vi "TetrisLV.vi"(11 "Board Size":T1={"X"=10, "Y"=20}) -> ()   [LabVIEW 2017]
uses:
  Controls/Coordinates.ctl
  Controls/Moves.ctl
  Game Board_class/Game Board.lvclass
  Wall_class/Wall.lvclass
  Piece of Bricks_class/Piece of Bricks.lvclass
panel:
  in  "Sounds On/Off":bool caption="Sounds"
  in  "Music On/Off":bool caption="Music"
  in  "Tableau":u32[][](array[colorbox])
  in  "Bouton Stop":bool
  out "Screen":u32[][](array[colorbox])
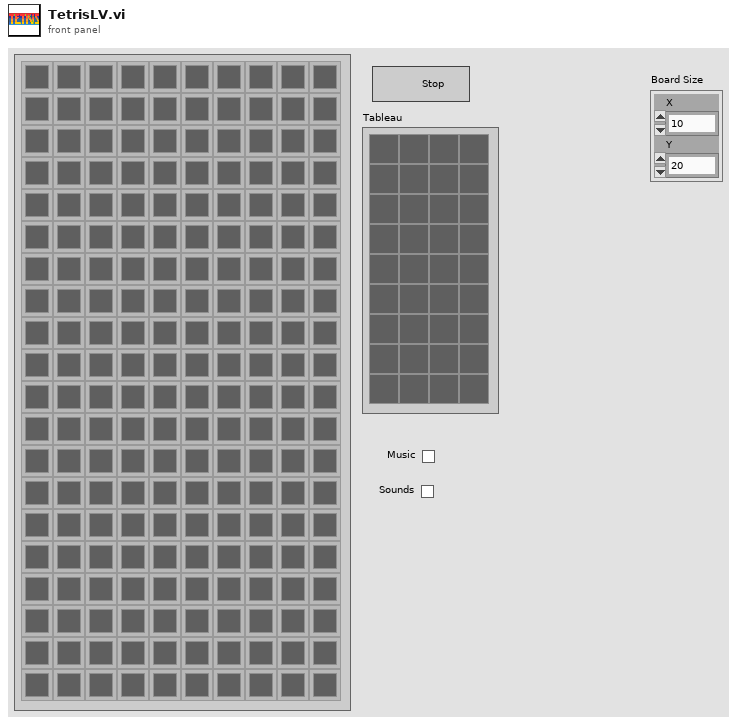
[diagram p1: front panel]
types:
  T1 = typedef "Coordinates.ctl" = cluster{"X":i32, "Y":i32}
  T2 = typedef "Moves.ctl" = enum16{"None", "Right", "Left", "Step Down", "Go Down", "90 Clockwise", "90 Anti-Clockwise"}
  T3 = enum32{"Invalid", "Standard", "Closed", "Hidden", "Minimized", "Maximized"}
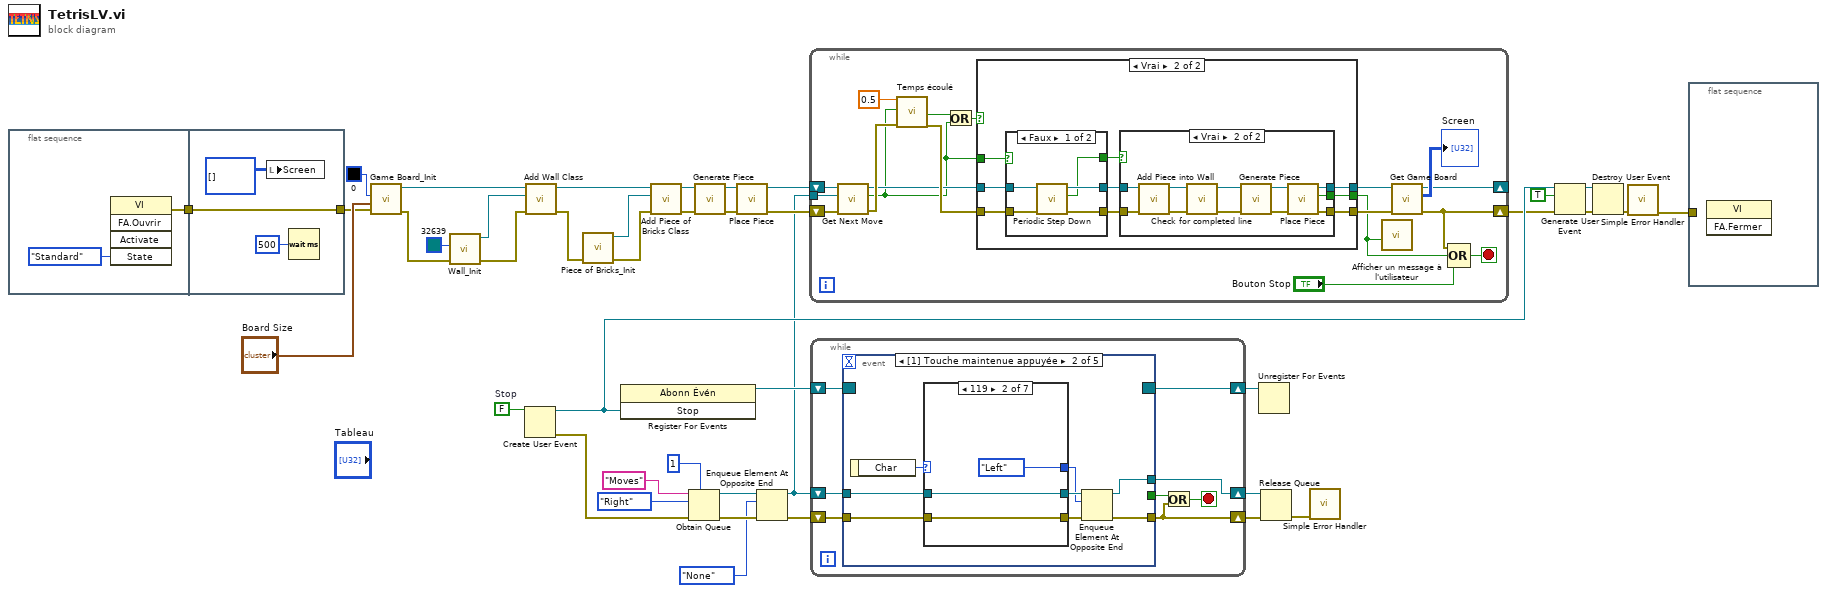
[diagram p0: block diagram]
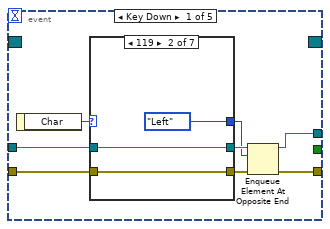
[diagram p2: hidden frame]
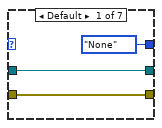
[diagram p3: hidden frame]
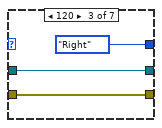
[diagram p4: hidden frame]
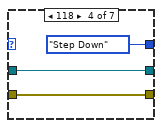
[diagram p5: hidden frame]
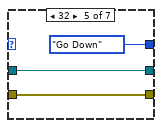
[diagram p6: hidden frame]
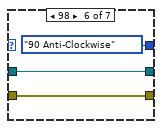
[diagram p7: hidden frame]
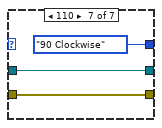
[diagram p8: hidden frame]
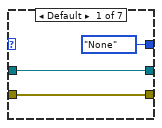
[diagram p9: hidden frame]
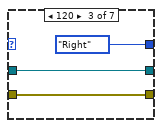
[diagram p10: hidden frame]
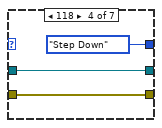
[diagram p11: hidden frame]
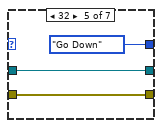
[diagram p12: hidden frame]
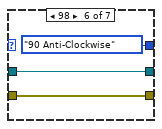
[diagram p13: hidden frame]
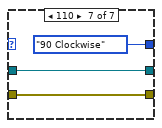
[diagram p14: hidden frame]
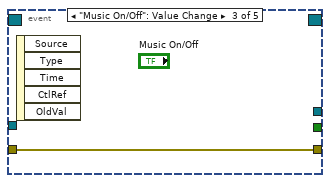
[diagram p15: hidden frame]
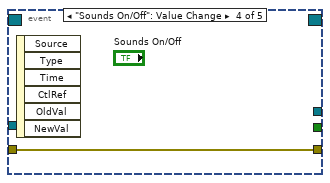
[diagram p16: hidden frame]
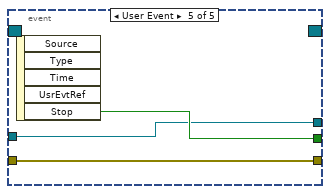
[diagram p17: hidden frame]
diagram:
  w38 = FALSE  # Stop
  n1 = flat-sequence {
    tunnel: [w42] -> w1
    tunnel: [w46] -> w2
    tunnel: w1 -> [w46]
    frame #0 {
      n2 = invoke class="VI" method="FA.Ouvrir"("State"=T3."Standard" ("État")) -> (error out=w42:errorcluster)  [unwired: 4 in, 4 out]
    }
    frame #1 {
      n3 = local write "Screen"(u32[][] []) -> ()
      n4 = Wait (ms)(milliseconds to wait=u32 500 ("attente (ms)")) -> ()  [unwired: 1 out]
    }
  }
  n5 = call "Game Board_Init.vi"("error in (no error)"=w2, "Board Size"="Board Size", "Board color"=u32 0) -> ("error out"=w28:errorcluster, "object out"=w11:refnum<class "Game Board.lvclass">)  [unwired: 7 in]
  n6 = call "Wall_Init.vi"("error in (no error)"=w28, "Wall Color"=u32 32639) -> ("error out"=w26:errorcluster, "object out"=w25:refnum<class "Wall.lvclass">)  [unwired: 8 in]
  n7 = Create User Event(user event datatype=w38) -> (user event=w35:refnum<user-event>, error out=w37:errorcluster)  [unwired: 1 in]
  n8 = call-dynamic "Add Wall Class.vi"("error in (no error)"=w26, "WallRef"=w25, "object in"=w11) -> ("error out"=w22:errorcluster, "object out"=w21:refnum<class "Game Board.lvclass">)  [unwired: 7 in]
  n9 = call "Piece of Bricks_Init.vi"("error in (no error)"=w22) -> ("error out"=w19:errorcluster, "object out"=w18:refnum<class "Piece of Bricks.lvclass">)  [unwired: 9 in]
  n10 = register-events(w35) -> (reference out=w36:refnum<event-registration>)  [unwired: 2 in, 1 out]
  n11 = call-dynamic "Add Piece of Bricks Class.vi"("error in (no error)"=w19, "Piece of Bricks"=w18, "object in"=w21) -> ("error out"=w20:errorcluster, "object out"=w16:refnum<class "Game Board.lvclass">)  [unwired: 7 in]
  n12 = Obtain Queue(max queue size (-1, unlimited)=1 ("taille max de la file d'attente (-1, non limitée)"), name (unnamed)="Moves" ("nom (aucun)"), element data type=Moves."Right" ("Enum"), error in (no error)=w37) -> (queue out=w8:refnum<queue>, error out=w39:errorcluster)  [unwired: 1 in, 1 out]
  n13 = call-dynamic "Generate Piece.vi"("error in (no error)"=w20, "Game Board en entrée"=w16) -> ("error out"=w17:errorcluster, "Game Board en sortie"=w10:refnum<class "Game Board.lvclass">)  [unwired: 8 in]
  n14 = call-dynamic "Place Piece.vi"("error in (no error)"=w17, "Game Board en entrée"=w10) -> ("error out"=w15:errorcluster, "Game Board en sortie"=w14:refnum<class "Game Board.lvclass">)  [unwired: 7 in, 1 out]
  n15 = Enqueue Element At Opposite End(queue=w8, element=Moves."None" ("élément"), error in (no error)=w39) -> (queue out=w7:refnum<queue>, error out=w9:errorcluster)  [unwired: 1 in, 1 out]
  n16 = while {
    tunnel: w7 -> [w60]
    shift-right: [w55] -> w31
    shift-left: w15 -> [w62]
    shift-right: [w58] -> _
    shift-left: w14 -> [w61]
    stop <- w63 stop-if-true
    n17 = call-dynamic "Get Next Move.vi"("error in (no error)"=w62, "Move queue"=w60, "Game Board en entrée"=w61) -> ("error out"=w53:errorcluster, "Freeze Piece"=w47:bool, "Game Board en sortie"=w51:refnum<class "Game Board.lvclass">)  [unwired: 6 in]
    n18 = call "Temps écoulé"("Time Target (s)"=0.5, "Reset"=w47, "error in (no error)"=w53) -> ("Time has Elapsed"=w50:bool, "error out"=w52:errorcluster)  [unwired: 9 in, 6 out]
    n19 = Or(x=w50, y=w47) -> (x .or. y?=w48:bool)
    n20 = case shown="Vrai" w48 {
      tunnel: [w66 w70] -> w57
      tunnel: [w65 w69] -> w56
      tunnel: w52 -> [w65 w75]
      tunnel: w51 -> [w66 w74]
      tunnel: w47 -> [_ w73]
      tunnel: [_ w67] -> w54
      frame False {
      }
      frame True {
        n21 = case shown="Faux" w73 {
          selector: w73 -> [_ w94]
          tunnel: [w93 w96] -> w71
          tunnel: [w92 w95] -> w68
          tunnel: w75 -> [w91 w95]
          tunnel: w74 -> [w90 w96]
          tunnel: [w89 w94] -> w72
          frame False {
            n22 = call-dynamic "Periodic Step Down.vi"("error in (no error)"=w91, "Game Board en entrée"=w90) -> ("error out"=w92:errorcluster, "Freeze Piece"=w89:bool, "Game Board en sortie"=w93:refnum<class "Game Board.lvclass">)  [unwired: 7 in]
          }
          frame True {
          }
        }
        n23 = case shown="Vrai" w72 {
          tunnel: [w76 w83] -> w70
          tunnel: w71 -> [w76 w88]
          tunnel: [w77 w85] -> w69
          tunnel: w68 -> [w77 w87]
          tunnel: [_ w82] -> w67
          frame False {
          }
          frame True {
            n24 = call-dynamic "Add Piece into Wall.vi"("error in (no error)"=w87, "Game Board en entrée"=w88) -> ("error out"=w80:errorcluster, "Game Board en sortie"=w81:refnum<class "Game Board.lvclass">)  [unwired: 8 in]
            n25 = call-dynamic "Check for completed line.vi"("error in (no error)"=w80, "Game Board en entrée"=w81) -> ("error out"=w78:errorcluster, "Game Board en sortie"=w79:refnum<class "Game Board.lvclass">)  [unwired: 8 in]
            n26 = call-dynamic "Generate Piece.vi"("error in (no error)"=w78, "Game Board en entrée"=w79) -> ("error out"=w86:errorcluster, "Game Board en sortie"=w84:refnum<class "Game Board.lvclass">)  [unwired: 8 in]
            n27 = call-dynamic "Place Piece.vi"("error in (no error)"=w86, "Game Board en entrée"=w84) -> ("error out"=w85:errorcluster, "Board Full"=w82:bool, "Game Board en sortie"=w83:refnum<class "Game Board.lvclass">)  [unwired: 7 in]
          }
        }
      }
    }
    n28 = call "Afficher un message à l'utilisateur"("Enable"=w54) -> ()  [unwired: 9 in, 2 out]
    n29 = call-dynamic "Get Game Board.vi"("error in (no error)"=w56, "Game Board en entrée"=w57) -> ("error out"=w55:errorcluster, "Game Board"=→"Screen":u32[][], "Game Board en sortie"=w58:refnum<class "Game Board.lvclass">)  [unwired: 7 in]
    n30 = Compound Arithmetic op=OR ("Opérateur arithmétique")(w55, w54, "Bouton Stop") -> (w63:bool)
  }
  n31 = while {
    shift-right: [w101] -> w24
    shift-left: w9 -> [w104]
    shift-right: [w97] -> w23
    shift-left: w7 -> [w103]
    shift-right: [w98] -> w30
    shift-left: w36 -> [w102]
    stop <- w99 stop-if-true
    n32 = event shown="[1] Touche maintenue appuyée" {
      selector: w102 -> [_ _ _ _ _]
      dyn-events: [_ _ _ _ _] -> w98
      timeout: _ -> [_ _ _ _ _]
      tunnel: w104 -> [w110 w139 w163 w164 w167]
      tunnel: w103 -> [w111 w140 _ _ w165]
      tunnel: [w108 w137 w163 w164 w167] -> w101
      tunnel: [_ _ _ _ w166] -> w100
      tunnel: [w105 w134 _ _ w165] -> w97
      event Key Down {
        n33 = event-data() -> ("Char"=w112:i16)  [unwired: 1 in]
        n34 = case shown="119" w112 {
          tunnel: w111 -> [w114 w117 w120 w123 w126 w129 w132]
          tunnel: w110 -> [w115 w118 w121 w124 w127 w130 w133]
          tunnel: [w115 w118 w121 w124 w127 w130 w133] -> w109
          tunnel: [w114 w117 w120 w123 w126 w129 w132] -> w107
          tunnel: [Moves."None" ("Enum") Moves."Left" ("Enum") Moves."Right" ("Enum") Moves."Step Down" ("Enum") Moves."Go Down" ("Enum") Moves."90 Anti-Clockwise" ("Enum") Moves."90 Clockwise" ("Enum")] -> w106
          frame Default {
          }
          frame 119 {
          }
          frame 120 {
          }
          frame 118 {
          }
          frame 32 {
          }
          frame 98 {
          }
          frame 110 {
          }
        }
        n35 = Enqueue Element At Opposite End(queue=w107, element=w106, error in (no error)=w109) -> (queue out=w105:refnum<queue>, error out=w108:errorcluster)  [unwired: 1 in, 1 out]
      }
      event Key Repeat {
        n36 = event-data() -> ("Char"=w141:i16)  [unwired: 1 in]
        n37 = case shown="119" w141 {
          tunnel: w140 -> [w143 w146 w149 w152 w155 w158 w161]
          tunnel: w139 -> [w144 w147 w150 w153 w156 w159 w162]
          tunnel: [w144 w147 w150 w153 w156 w159 w162] -> w138
          tunnel: [w143 w146 w149 w152 w155 w158 w161] -> w136
          tunnel: [Moves."None" ("Enum") Moves."Left" ("Enum") Moves."Right" ("Enum") Moves."Step Down" ("Enum") Moves."Go Down" ("Enum") Moves."90 Anti-Clockwise" ("Enum") Moves."90 Clockwise" ("Enum")] -> w135
          frame Default {
          }
          frame 119 {
          }
          frame 120 {
          }
          frame 118 {
          }
          frame 32 {
          }
          frame 98 {
          }
          frame 110 {
          }
        }
        n38 = Enqueue Element At Opposite End(queue=w136, element=w135, error in (no error)=w138) -> (queue out=w134:refnum<queue>, error out=w137:errorcluster)  [unwired: 1 in, 1 out]
      }
      event "Music On/Off": Value Change {
        n39 = event-data() -> ()  [unwired: 1 in, 5 out]
      }
      event "Sounds On/Off": Value Change {
        n40 = event-data() -> ()  [unwired: 1 in, 6 out]
      }
      event User Event {
        n41 = event-data() -> ("Stop"=w166:bool)  [unwired: 1 in, 4 out]
      }
    }
    n42 = Or(x=w100, y=w101) -> (x .or. y?=w99:bool)
  }
  n43 = Unregister For Events(event registration refnum=w30) -> ()  [unwired: 1 in, 1 out]
  n44 = Release Queue(queue=w23, error in (no error)=w24) -> (error out=w12:errorcluster)  [unwired: 1 in, 2 out]
  n45 = call <vilib>:"Simple Error Handler.vi"("error in (no error)"=w12) -> ()  [unwired: 4 in, 5 out]
  n46 = Generate User Event(user event=w35, event data cluster=TRUE ("données d'événement"), error in=w31) -> (user event out=w33:refnum<user-event>, error out=w34:errorcluster)  [unwired: 1 in]
  n47 = Destroy User Event(user event=w33, error in=w34) -> (error out=w13:errorcluster)
  n48 = call <vilib>:"Simple Error Handler.vi"("error in (no error)"=w13) -> ("error out"=w5:errorcluster)  [unwired: 4 in, 4 out]
  n49 = flat-sequence {
    tunnel: w5 -> [_]
    frame #0 {
      n50 = invoke class="VI" method="FA.Fermer"() -> ()  [unwired: 3 in, 3 out]
    }
  }
